vi "Variable@Shift__Parameter.vi"(1 "ParamterIn":string) -> (0 "ParamterOut":string)   [LabVIEW 2020]
panel:
  out "Key":string[](array[string])
  in  "Section":string(combo)
  in  "Shift":string(combo)
  in  "Var1":string(combo)
  in  "Confirm":bool
  # "Variable@Shift $Variable1,$Vairable2.......(,Shift=X,Section=X)"
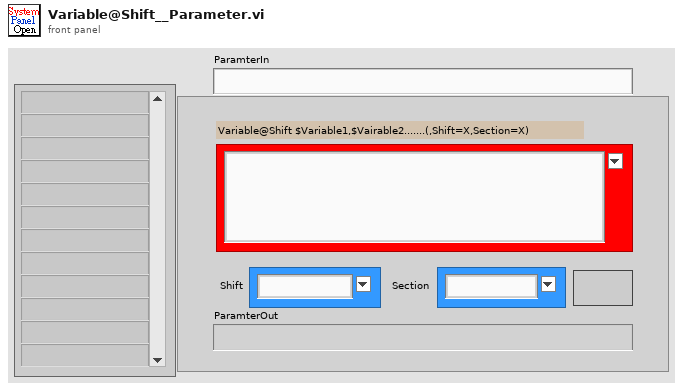
[diagram p1: front panel]
types:
  T1 = enum16{"Get", "Init", "Set", "Delete", "GetElement", "Inc", "Dec", "ReName"}
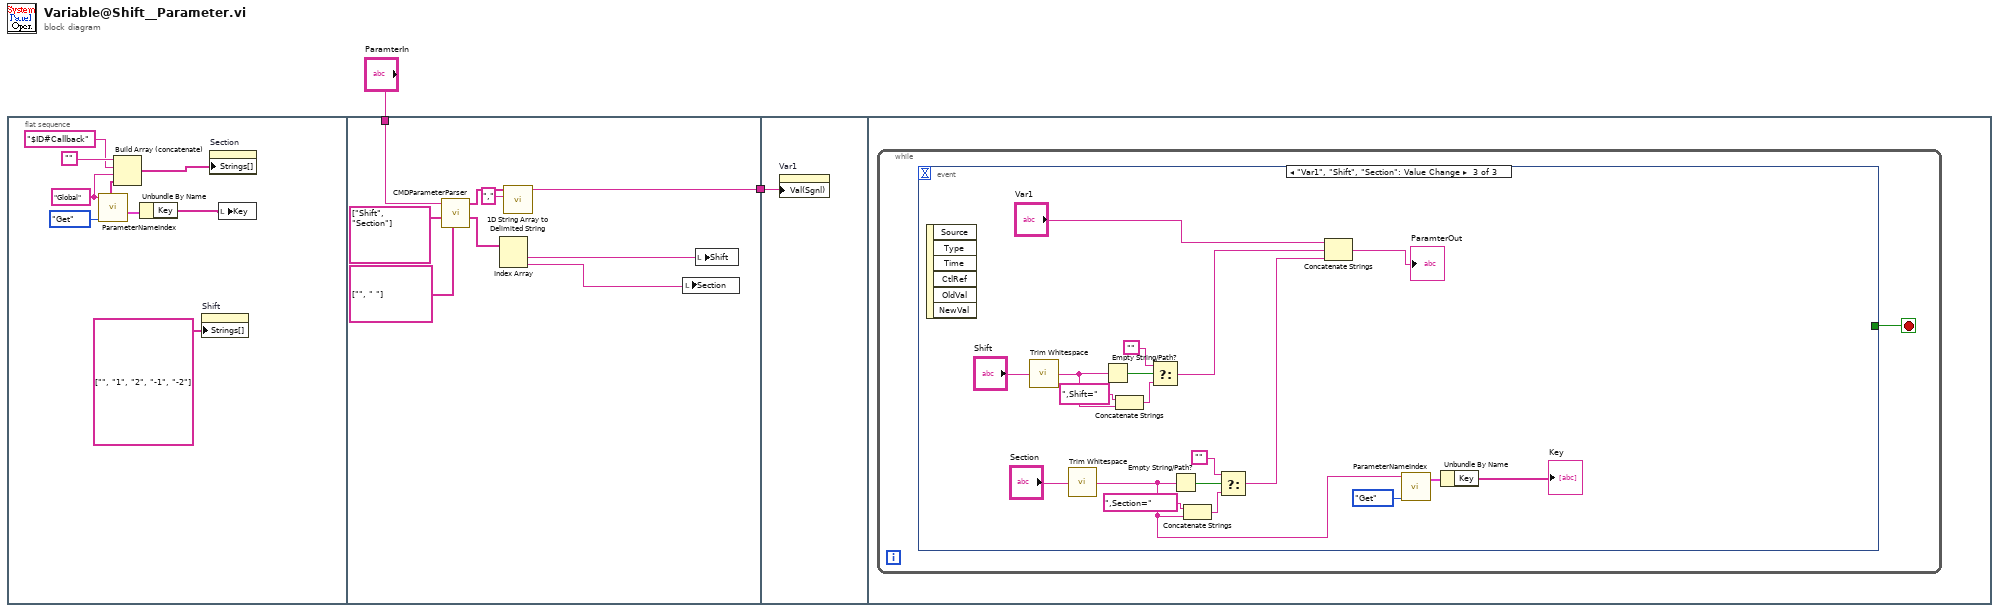
[diagram p0: block diagram]
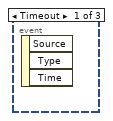
[diagram p2: hidden frame]
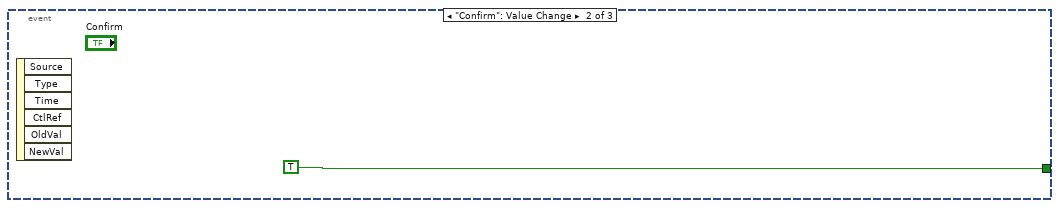
[diagram p3: hidden frame]
diagram:
  n1 = flat-sequence {
    tunnel: "ParamterIn" -> [w20]
    tunnel: [w15] -> w1
    tunnel: w1 -> [w21]
    frame #0 {
      w7 = "Global" ("VariableSection")
      n2 = call "ParameterNameIndex.vi"("OP"=T1."Get", "VariableSection"=w7) -> ("GlobalKeyValue"=w11:cluster{"Key":string[], "Value":string[]}, "SectionList"=w8:string[])  [unwired: 3 in, 5 out]
      n3 = Build Array (concatenate)("", "$ID#Callback" ("VariableSection"), w7, w8) -> (w6:string[])
      n4 = Unbundle By Name(w11) -> ("Key"=w3:string[])
      n5 = property on="Shift" class="CmbBox"("Strings[]"=string[] ["", "1", "2", "-1", "-2"] ("Strings []")) -> ()  [unwired: 2 in, 2 out]
      n6 = property on="Section" class="CmbBox"("Strings[]"=w6) -> ()  [unwired: 2 in, 2 out]
      n7 = local write "Key"(w3) -> ()
    }
    frame #1 {
      n8 = call "CMDParameterParser.vi"("DeafultValues"=string[] ["", " "], "RequiredKeys"=string[] ["Shift", "Section"], "CMDParameter"=w20) -> ("KeyValues"=w14:string[], "Input"=w17:string[])  [unwired: 6 in, 1 out]
      n9 = Index Array(array=w14) -> (element #1=w13:string, element #2=w12:string)  [unwired: 2 in]
      n10 = call <vilib>:"1D String Array to Delimited String.vi"("delimiter"=",", "string array"=w17) -> ("delimited string"=w15:string)  [unwired: 9 in]
      n11 = local write "Section"(w12) -> ()
      n12 = local write "Shift"(w13) -> ()
    }
    frame #2 {
      n13 = property on="Var1" class="CmbBox"("Val(Sgnl)"=w21) -> ()  [unwired: 2 in, 2 out]
    }
    frame #3 {
      n14 = while {
        stop <- w22 stop-if-true
        n15 = event shown="[2] \"Var1\", \"Shift\", \"Section\": Value Change" {
          selector: _ -> [_ _ _]
          dyn-events: _ -> [_ _ _]
          timeout: _ -> [_ _ _]
          tunnel: [_ TRUE _] -> w22
          event Timeout {
            n16 = event-data() -> ()  [unwired: 1 in, 3 out]
          }
          event "Confirm": Value Change {
            n17 = event-data() -> ()  [unwired: 1 in, 6 out]
          }
          event "Var1", "Shift", "Section": Value Change {
            n18 = event-data() -> ()  [unwired: 1 in, 6 out]
            n19 = call <vilib>:"Trim Whitespace.vi"("string"="Shift") -> ("trimmed string"=w24:string)  [unwired: 1 in]
            n20 = call <vilib>:"Trim Whitespace.vi"("string"="Section") -> ("trimmed string"=w26:string)  [unwired: 1 in]
            n21 = Empty String/Path?(string/path=w24) -> (empty?=w33:bool)
            n22 = Concatenate Strings(",Shift=" ("string"), w24) -> (w32:string)
            n23 = Select(t="", s=w33, f=w32) -> (s? t:f=w30:string)
            n24 = Empty String/Path?(string/path=w26) -> (empty?=w38:bool)
            n25 = Concatenate Strings(",Section=" ("string"), w26) -> (w39:string)
            n26 = Select(t="", s=w38, f=w39) -> (s? t:f=w29:string)
            n27 = Concatenate Strings("Var1", w30, w29) -> (→"ParamterOut":string)
            n28 = call "ParameterNameIndex.vi"("OP"=T1."Get", "VariableSection"=w26) -> ("SectionKeyValue"=w35:cluster{"Key":string[], "Value":string[]})  [unwired: 3 in, 6 out]
            n29 = Unbundle By Name(w35) -> ("Key"=→"Key":string[])
          }
        }
      }
    }
  }
